vi "execute.vi"(8 "error in (no error)":errorcluster, 9 "DAQ in (B)":refnum<class "GenericComponent.lvclass">, 10 "ImagingMode in (A)":refnum<class "GenericComponent.lvclass">, 11 "AdapterMH110616ImagingModeToDAQ in":refnum<class "AdapterMH110616ImagingModeToDAQ.lvclass">) -> (0 "error out":errorcluster, 1 "DAQ out (B)":refnum<class "GenericComponent.lvclass">, 2 "ImagingMode out (A)":refnum<class "GenericComponent.lvclass">, 3 "AdapterMH110616ImagingModeToDAQ out":refnum<class "AdapterMH110616ImagingModeToDAQ.lvclass">)   [LabVIEW 2010, in "AdapterMH110616ImagingModeToDAQ.lvclass"]
uses:
  AdapterMH110616ImagingModeToDAQ.lvclass
  common/classes/GenericComponent/GenericComponent/GenericComponent.lvclass
  ImagingMode/ImagingModeDL090130Frame/ImagingModeDL090130Frame/ImagingModeDL090130Frame.lvclass
  DAQ/DAQ_MG090622Camera/DAQ_MG090622Camera/DAQ_MG090622Camera.lvclass
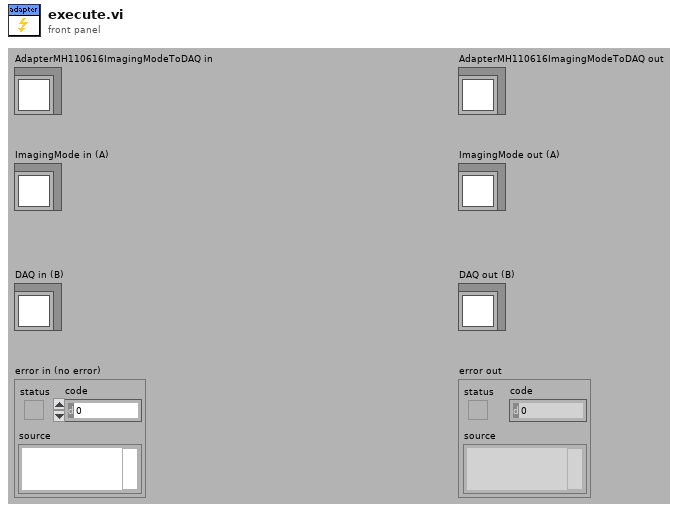
[diagram p1: front panel]
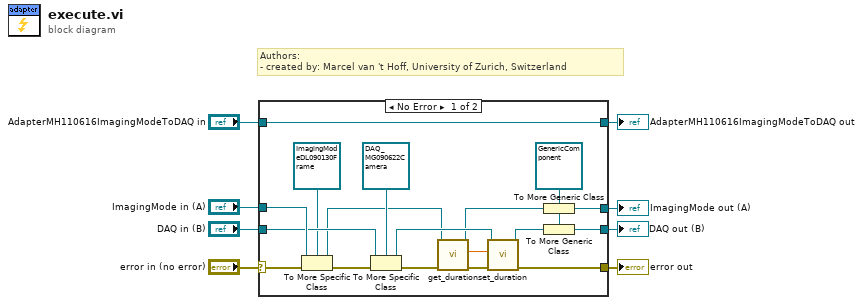
[diagram p0: block diagram]
diagram:
  # "Authors: \n- created by: Marcel van 't Hoff, University of Zurich, Switzerland"
  n1 = case shown="No Error" "error in (no error)" {
    selector: "error in (no error)" -> [w21 w29]
    tunnel: [w20 w29] -> w7
    tunnel: "DAQ in (B)" -> [w23 w28]
    tunnel: "ImagingMode in (A)" -> [w25 w27]
    tunnel: "AdapterMH110616ImagingModeToDAQ in" -> [w26 w30]
    tunnel: [w26 w30] -> w3
    tunnel: [w16 w27] -> w2
    tunnel: [w15 w28] -> w1
    frame No Error {
      w17 = refnum<class "GenericComponent.lvclass"> refnum ("GenericComponent.lvclass")
      n2 = To More Specific Class(target class=refnum<class "ImagingModeDL090130Frame.lvclass"> refnum ("ImagingModeDL090130Frame.lvclass"), reference=w25, error in=w21) -> (specific class reference=w9:refnum<class "ImagingModeDL090130Frame.lvclass">, error out=w22:errorcluster)
      n3 = To More Specific Class(target class=refnum<class "DAQ_MG090622Camera.lvclass"> refnum ("DAQ_MG090622Camera.lvclass"), reference=w23, error in=w22) -> (specific class reference=w19:refnum<class "DAQ_MG090622Camera.lvclass">, error out=w10:errorcluster)
      n4 = call-dynamic "get_duration.vi"("error in (no error)"=w10, "ImagingModeDL090130Frame in"=w9) -> ("error out"=w11:errorcluster, "duration"=w12:dbl[unit], "ImagingModeDL090130Frame out"=w13:refnum<class "ImagingModeDL090130Frame.lvclass">)  [unwired: 7 in]
      n5 = call-dynamic "set_duration.vi"("error in (no error)"=w11, "duration"=w12, "DAQ_MG090622Camera in"=w19) -> ("error out"=w20:errorcluster, "DAQ_MG090622Camera out"=w18:refnum<class "DAQ_MG090622Camera.lvclass">)  [unwired: 7 in]
      n6 = To More Generic Class(target class=w17, reference=w13) -> (generic class reference=w16:refnum<class "GenericComponent.lvclass">)
      n7 = To More Generic Class(target class=w17, reference=w18) -> (generic class reference=w15:refnum<class "GenericComponent.lvclass">)
    }
    frame Error {
    }
  }
  "error out" <- w7
  "AdapterMH110616ImagingModeToDAQ out" <- w3
  "ImagingMode out (A)" <- w2
  "DAQ out (B)" <- w1
